vi "Phase subtract.vi"(7 "unwrap phase":bool, 9 "previous phase":dbl[](array[numeric]), 10 "phase ref":dbl[](array[numeric]), 11 "Phase in":dbl[][](array[numeric])) -> (1 "last phase":dbl[](array[numeric]), 3 "Phase out":dbl[][](array[numeric]))   [LabVIEW 2018]
uses:
  <vilib>/Analysis/coordinate.llb/Angle Units.ctl
  <vilib>/Analysis/NI_AAL_Angle.lvlib
  <vilib>/Analysis/NI_AALPro.lvlib
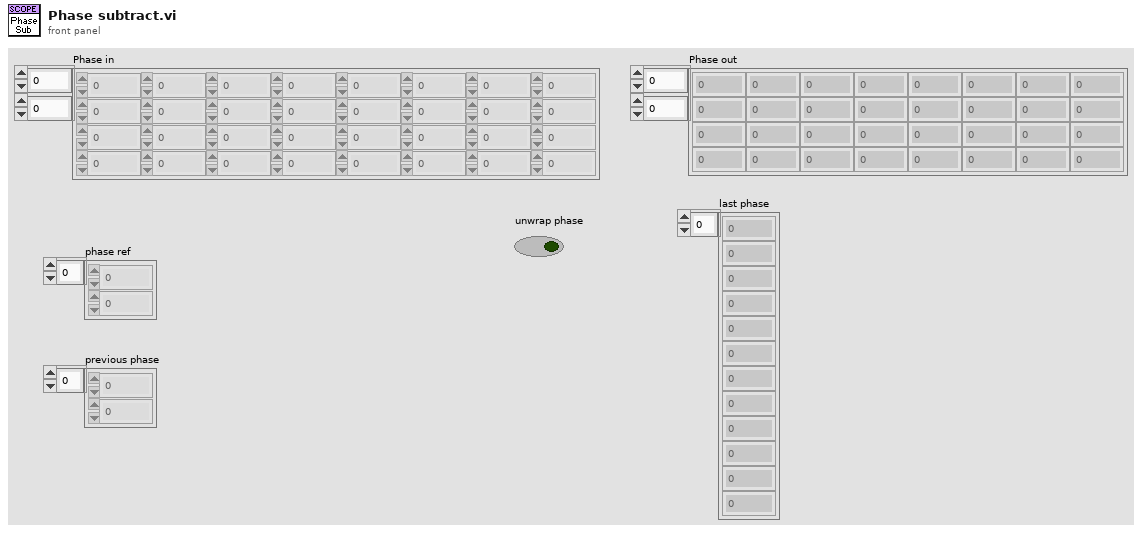
[diagram p1: front panel]
types:
  T1 = typedef "NI_AAL_Angle.lvlib/Angle Units.ctl" = i32
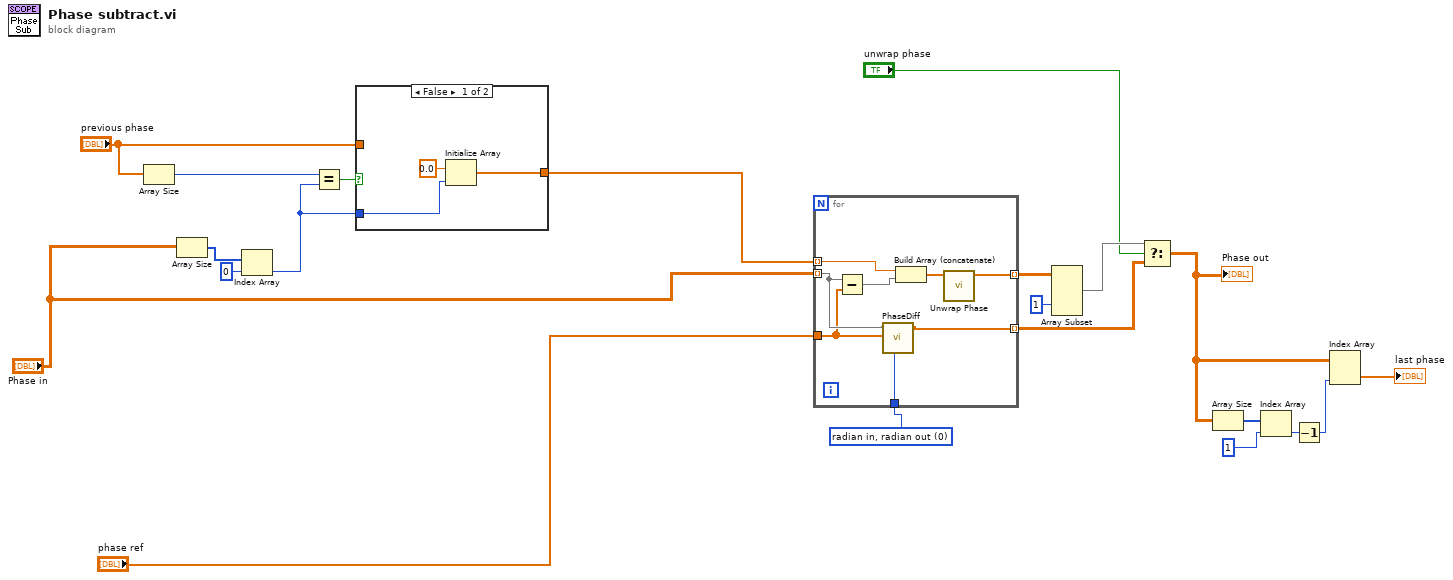
[diagram p0: block diagram]
diagram:
  w14 = T1 0 items=["radian in, radian out", "radian in, degree out", "degree in, degree out", "degree in, radian out"] ("angle units")
  n1 = Array Size(array="previous phase") -> (size(s)=w13:i32)
  n2 = Array Size(array="Phase in") -> (size(s)=w6:i32[])
  n3 = Index Array(array=w6, index=0) -> (element=w4:i32)
  n4 = Equal?(x=w13, y=w4) -> (x = y?=w12:bool)
  n5 = case shown="False" w12 {
    tunnel: "previous phase" -> [_ w25]
    tunnel: [w22 w25] -> w2
    tunnel: w4 -> [w23 _]
    frame False {
      n6 = Initialize Array(0.0 ("element"), w23) -> (w22:dbl[])
    }
    frame True {
    }
  }
  n7 = for {
    tunnel: "Phase in" -> [w29] mode=indexing
    tunnel: "phase ref" -> [w28]
    tunnel: [w33] -> w15 mode=indexing
    tunnel: w2 -> [w32] mode=indexing
    tunnel: [w27] -> w8 mode=indexing
    tunnel: w14 -> [w26]
    n8 = Subtract(x=w29, y=w28) -> (x-y=w30:dbl[])
    n9 = call "PhaseDiff.vi"("angle units"=w26, "Angle 2"=w28, "Angle 1"=w29) -> ("Absolute Angle Difference"=w27:dbl[])  [unwired: 5 in]
    n10 = Build Array (concatenate)(w32, w30) -> (w31:dbl[])
    n11 = call <vilib>:"Unwrap Phase.vi"("Phase"=w31) -> ("Unwrapped Phase"=w33:dbl[])  [unwired: 9 in, 1 out]
  }
  n12 = Array Subset(array=w15, index (col)=1 ("index")) -> (w10:dbl[][])  [unwired: 3 in]
  n13 = Select(t=w10, s="unwrap phase", f=w8) -> (s? t:f=w9:dbl[][])
  "Phase out" <- w9
  n14 = Array Size(array=w9) -> (size(s)=w21:i32[])
  n15 = Index Array(array=w21, index=1) -> (element=w20:i32)
  n16 = Decrement(x=w20) -> (x-1=w18:i32)
  n17 = Index Array(array=w9, index (col)=w18) -> (element=→"last phase":dbl[])  [unwired: 1 in]
